vi "Between 2 angles.vi"(8 "Test Angle":dbl, 10 "Angle 2":dbl, 11 "Angle 1":dbl) -> (3 "Is between Angle 1 and Angle 2":bool)   [LabVIEW 2012]
panel:
  out "coerced(x)":dbl
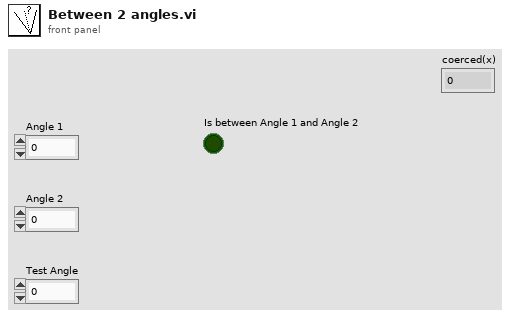
[diagram p1: front panel]
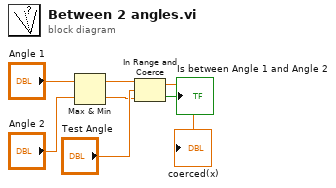
[diagram p0: block diagram]
diagram:
  n1 = Max & Min(x="Angle 1", y="Angle 2") -> (max(x,y)=w3:dbl, min(x,y)=w2:dbl)
  n2 = In Range and Coerce(upper limit=w3, x="Test Angle", lower limit=w2) -> (coerced(x)=→"coerced(x)":dbl, In Range?=→"Is between Angle 1 and Angle 2":bool)
